vi "FCO_Zero.vi"(8 "错误输入（无错误）":errorcluster caption="Error in", 11 "VISA in":refnum<visa-resource-name>) -> (0 "错误输出":errorcluster caption="Error out", 2 "data":string, 3 "VISA out":refnum<visa-resource-name>)   [LabVIEW 2017]
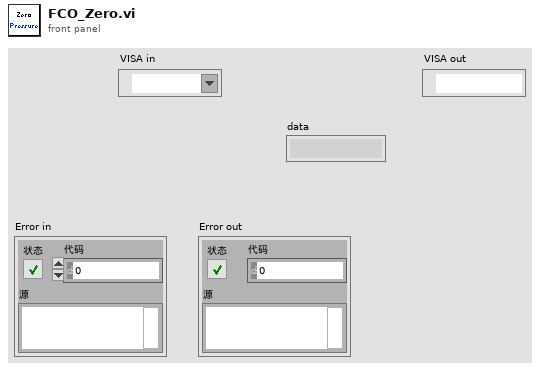
[diagram p1: front panel]
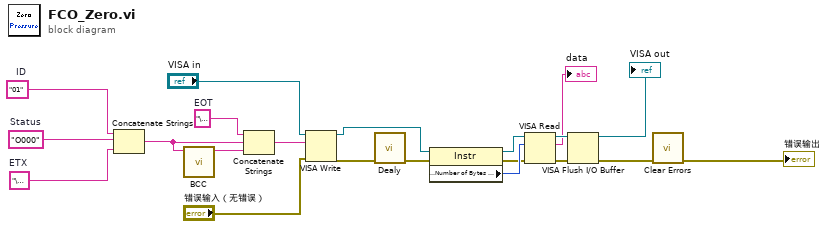
[diagram p0: block diagram]
diagram:
  w2 = "01"  # ID
  w5 = "\u0003"  # ETX
  w7 = "O000"  # Status
  w19 = "\u0004"  # EOT
  n1 = Concatenate Strings(w2, w7, w5) -> (w20:string)
  n2 = call "BCC.vi"("输入校验十六进制"=w20) -> ("BCC校验结果"=w21:string)  [unwired: 10 in]
  n3 = Concatenate Strings(w19, w20, w21) -> (w18:string)
  n4 = VISA Write(VISA resource name="VISA in", write buffer=w18, error in (no error)="错误输入（无错误）") -> (VISA resource name out=w10:refnum<visa-resource-name>, error out=w11:errorcluster)  [unwired: 1 out]
  n5 = call "Dealy"("error in (no error)"=w11) -> ("error out"=w16:errorcluster)  [unwired: 10 in]
  n6 = property class="Instr"(reference=w10, error in=w16) -> (reference out=w12:refnum<visa-resource-name>, error out=w13:errorcluster, "Serial Settings:Number of Bytes at Serial Port"=w14:u32)
  n7 = VISA Read(VISA resource name=w12, byte count=w14, error in (no error)=w13) -> (VISA resource name out=w17:refnum<visa-resource-name>, read buffer=→"data":string, error out=w15:errorcluster)  [unwired: 1 out]
  n8 = VISA Flush I/O Buffer(VISA resource name=w17, error in (no error)=w15) -> (VISA resource name out=→"VISA out":refnum<visa-resource-name>, error out=w9:errorcluster)  [unwired: 1 in]
  n9 = call <vilib>:"Clear Errors.vi"("error in (no error)"=w9) -> ("error out"=→"错误输出":errorcluster)  [unwired: 5 in, 1 out]
